vi "setUp.vi"(8 "error in (no error)":errorcluster, 11 "reference in":refnum<class "Pass If Equal Timestamp Test Case.lvclass">) -> (0 "error out":errorcluster, 3 "reference out":refnum<class "Pass If Equal Timestamp Test Case.lvclass">)   [LabVIEW 2015, in "Pass If Equal Timestamp Test Case.lvclass"]
doc: "setUp runs prior to the test method during test execution. Use this method to initialize any object data required by your tests."
uses:
  Pass If Equal Timestamp Test Case.lvclass
  Pass If Equal Timestamp Test Case.lvclass/Pass If Equal Timestamp Test Case.ctl
  <vilib>/addons/_JKI Toolkits/VI Tester/TestCase.llb/TestCase.lvclass
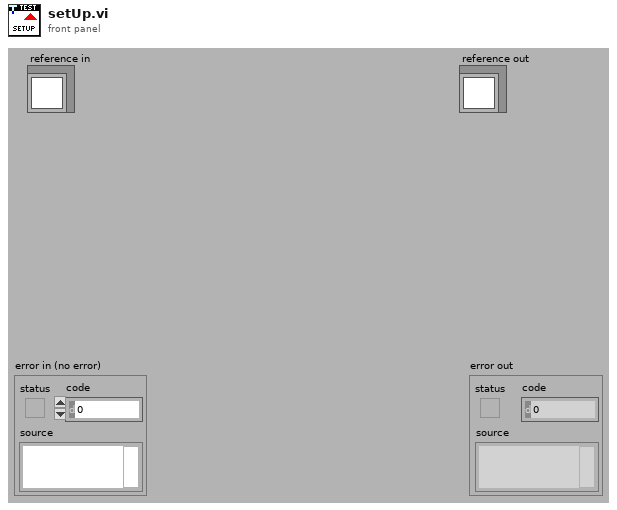
[diagram p1: front panel]
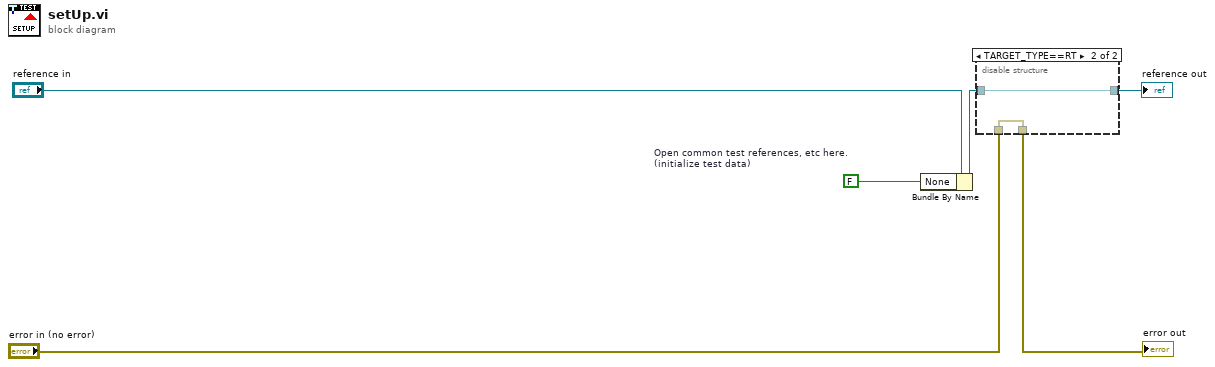
[diagram p0: block diagram]
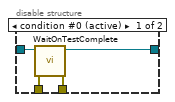
[diagram p2: hidden frame]
diagram:
  w1 = FALSE  # Open common test references, etc here. (initialize test data)
  n1 = Bundle By Name(cluster="reference in", "None"=w1) -> (w2:refnum<class "Pass If Equal Timestamp Test Case.lvclass">)
  n2 = disable-structure shown="TARGET_TYPE==RT" {
    disable-tunnel: "error in (no error)" -> [w10 w11]
    disable-tunnel: [w9 w11] -> w5
    disable-tunnel: [w8 w12] -> w3
    disable-tunnel: w2 -> [w7 w12]
    frame condition #0 (active) {
      n3 = call <vilib>:"WaitOnTestComplete.vi"("error in (no error)"=w10, "TestCase in"=w7) -> ("error out"=w9:errorcluster, "TestCase out"=w8:refnum<class "Pass If Equal Timestamp Test Case.lvclass">)  [unwired: 8 in]
    }
    frame condition #1 {
    }
  }
  "error out" <- w5
  "reference out" <- w3
